vi "prepAO_focusalign.vi"(3 "srate":dbl=30000.0, 4 "waveforms":waveform(dbl)[][](array[waveform]), 5 "Device chans":T1(array[cluster]), 6 "bufferAO":i32) -> (0 "AOerrout":errorcluster[](array[cluster]), 1 "Terminal Name with Device Prefix":tag, 2 "aochanarrays":refnum<k21>[](array[refnum]))   [LabVIEW 2015]
uses:
  <vilib>/DAQmx/write.llb/DAQmx Write (Analog Wfm 1Chan NSamp).vi
  <vilib>/DAQmx/write.llb/DAQmx Write (Analog 1D Wfm NChan NSamp).vi
  <vilib>/DAQmx/create/channels.llb/DAQmx Create Channel (AO-Voltage-Basic).vi
  <vilib>/DAQmx/configure/timing.llb/DAQmx Timing (Sample Clock).vi
  <vilib>/DAQmx/miscellaneous.llb/DAQmx Fill In Error Info.vi
  <vilib>/DAQmx/configure/trigger.llb/DAQmx Start Trigger (Digital Edge).vi
panel:
  in  "error in 3":errorcluster caption="error in"
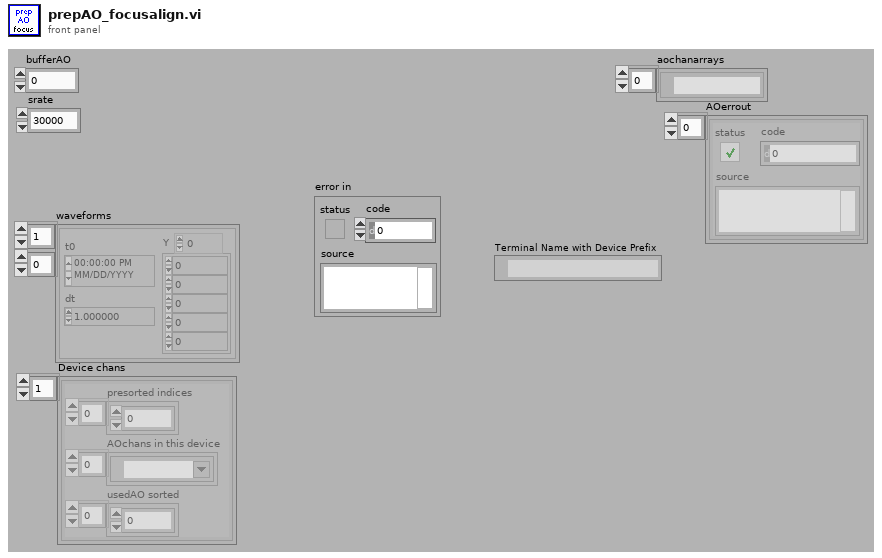
[diagram p1: front panel]
types:
  T1 = cluster{"presorted indices":i32[], "AOchans in this device":tag[], "usedAO sorted":i32[]}[]
  T2 = typedef "XYZStage.lvlib/XYZStage Configuration.ctl" = cluster{"VISA resource name":refnum<visa-resource-name>, "Timeout (3sec)":u32}
  T3 = cluster{"StageS":i32, "StageL":i32, "currmeas data dir":path, "image OD":u16, "contour OD":u16, "point OD":u16, "AOlines":tag[], "AIlines":tag[], "CI lines":tag[], "DO lines":tag[], "AO names":string[], "CI names":string[], "AI names":string[], "DO names":string[], "CIextensions":string[], "AIextensions":string[], "Voltage to Ygalvo":i32, "Voltage to Xgalvo":i32, "Voltage to patch":i32, "640 shutter":i32, "2P shutter":i32, "LT timestamp":u32, "Vp":i32, "Ip":i32, "camera trigger":i32, "master data dir":path, "voltage to Zpos":i32, "Vto2P":i32, "640 AO":i32, "488 AO":i32, "532 AO":i32, "640TTL":u32, "488TTL":u32, "532TTL":u32, "Device 1 sampleclock out":tag, "Device 1 Starttrigger out":tag, "Device 2 sampleclock in":tag, "Device 2 StartTrigger in ":tag, "2PODTTL":u32, "488 shutter":u32, "LCVR red":u32, "LCVR blue":u32, "Sutter Stage Config":T2}
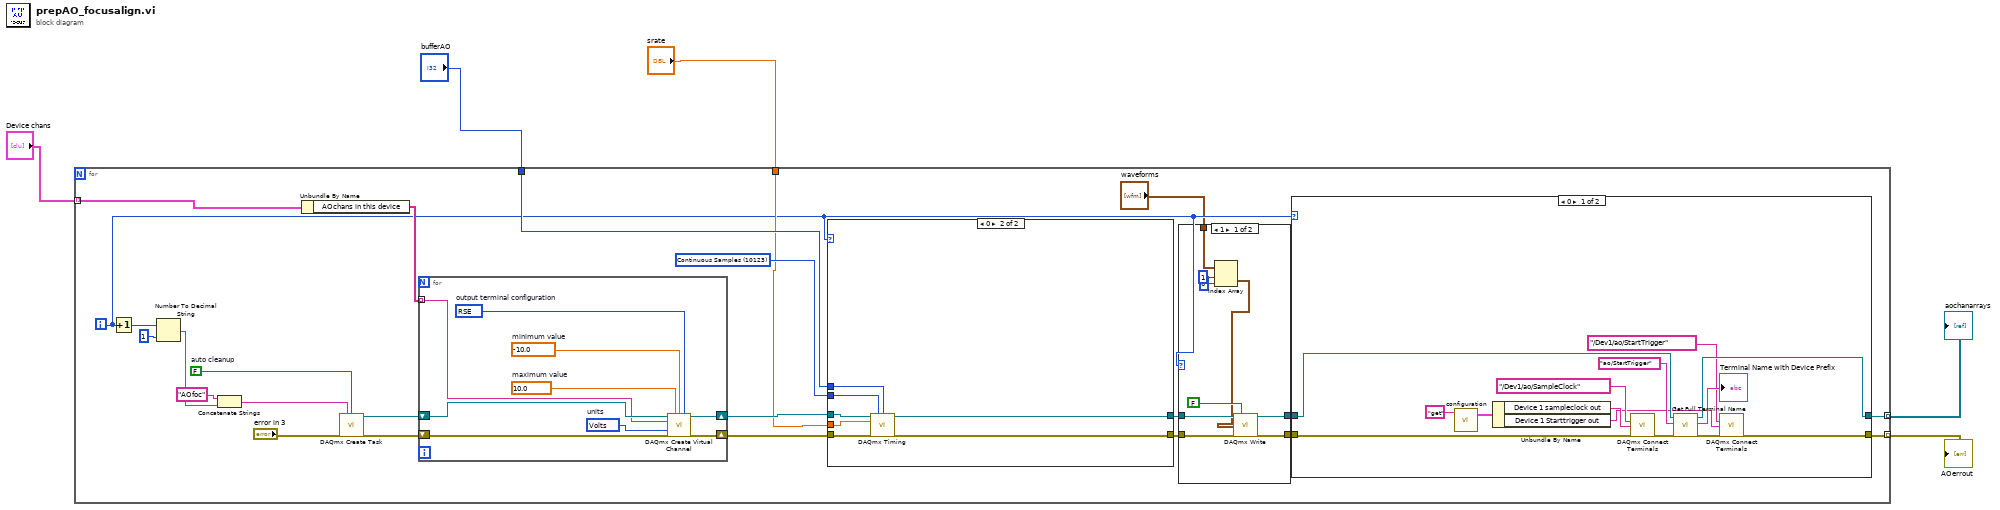
[diagram p0: block diagram]
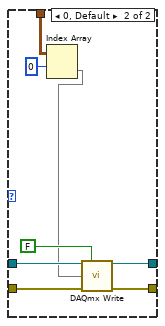
[diagram p2: hidden frame]
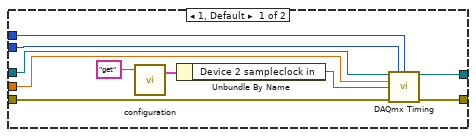
[diagram p3: hidden frame]
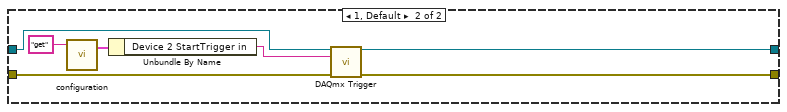
[diagram p4: hidden frame]
diagram:
  n1 = for {
    tunnel: "Device chans" -> [w23] mode=indexing
    tunnel: [w12] -> w5 mode=indexing
    tunnel: [w11] -> w4 mode=indexing
    tunnel: "bufferAO" -> [w9]
    tunnel: "srate" -> [w8]
    i -> [w7]
    w10 = 10123 items=["Finite Samples"=10178, "Continuous Samples"=10123, "Hardware Timed Single Point"=12522] ("sample mode")
    w27 = FALSE  # auto cleanup
    n2 = Increment(x=w7) -> (x+1=w20:i32)
    n3 = Number To Decimal String(number=w20, width (-)=i16 1) -> (decimal integer string=w19:string)
    n4 = Concatenate Strings("AOfoc" ("new task name"), w19) -> (w17:string)
    n5 = Unbundle By Name(w23) -> ("AOchans in this device"=w22:tag[])
    n6 = call <vilib>:"DAQmx Create Task.vi"("new task name"=w17, "auto cleanup"=w27, "error in"="error in 3") -> ("task out"=w28:refnum<k21>, "error out"=w29:errorcluster)  [unwired: 11 in]
    n7 = for {
      shift-right: [w87] -> w25
      shift-left: w28 -> [w89]
      shift-right: [w86] -> w24
      shift-left: w29 -> [w88]
      tunnel: w22 -> [w85] mode=indexing
      w93 = 10083 items=["Default"=-1, "RSE"=10083, "Differential"=10106, "Pseudodifferential"=12529]  # output terminal configuration
      w92 = 10348 items=["Volts"=10348, "From Custom Scale"=10065]  # units
      w91 = -10.0  # minimum value
      w90 = 10.0  # maximum value
      n8 = call-poly <vilib>:"DAQmx Create Virtual Channel.vi"("task in"=w89, "maximum value"=w90, "minimum value"=w91, "output terminal configuration"=w93, "physical channels"=w85, "units"=w92, "error in"=w88) -> ("task out"=w87:refnum<k21>, "error out"=w86:errorcluster)  [unwired: 7 in]
    }
    n9 = case shown="0" w7 {
      tunnel: w25 -> [w56 w63]
      tunnel: w24 -> [w55 w62]
      tunnel: w10 -> [w47 w61]
      tunnel: w8 -> [w54 w60]
      tunnel: w9 -> [w53 w59]
      tunnel: [w52 w58] -> w16
      tunnel: [w51 w57] -> w15
      frame 1, Default {
        n10 = call "configuration.vi"("command"="get") -> ("config out"=w49:T3)  [unwired: 2 in, 1 out]
        n11 = Unbundle By Name(w49) -> ("Device 2 sampleclock in"=w48:tag)
        n12 = call-poly <vilib>:"DAQmx Timing.vi"("task/channels in"=w56, "sample mode"=w47, "samples per channel"=w53, "rate"=w54, "source"=w48, "error in"=w55) -> ("task out"=w51:refnum<k21>, "error out"=w52:errorcluster)  [unwired: 1 in, 7 out]
      }
      frame 0 {
        n13 = call-poly <vilib>:"DAQmx Timing.vi"("task/channels in"=w63, "sample mode"=w61, "samples per channel"=w59, "rate"=w60, "error in"=w62) -> ("task out"=w57:refnum<k21>, "error out"=w58:errorcluster)  [unwired: 2 in, 7 out]
      }
    }
    n14 = case shown="1" w7 {
      tunnel: w16 -> [w37 w45]
      tunnel: w15 -> [w36 w44]
      tunnel: [w35 w43] -> w14
      tunnel: [w34 w42] -> w13
      tunnel: "waveforms" -> [w33 w41]
      frame 1 {
        n15 = Index Array(array=w33, index (row)=1, index (col)=0 ("disabled index (col)")) -> (element=w30:waveform(dbl))
        n16 = call-poly <vilib>:"DAQmx Write.vi"("task/channels in"=w36, "auto start"=FALSE, "data"=w30, "error in"=w37) -> ("task out"=w35:refnum<k21>, "error out"=w34:errorcluster)  [unwired: 9 in, 1 out]
      }
      frame 0, Default {
        n17 = Index Array(array=w41, index (row)=0) -> (element=w39:waveform(dbl)[])  [unwired: 1 in]
        n18 = call-poly <vilib>:"DAQmx Write.vi"("task/channels in"=w44, "auto start"=FALSE, "data"=w39, "error in"=w45) -> ("task out"=w43:refnum<k21>, "error out"=w42:errorcluster)  [unwired: 9 in, 1 out]
      }
    }
    n19 = case shown="0" w7 {
      tunnel: [w76 w84] -> w12
      tunnel: [w68 w83] -> w11
      tunnel: w13 -> [w72 w81]
      tunnel: w14 -> [w74 w82]
      frame 0 {
        n20 = call "configuration.vi"("command"="get") -> ("config out"=w67:T3)  [unwired: 2 in, 1 out]
        n21 = Unbundle By Name(w67) -> ("Device 1 sampleclock out"=w65:tag, "Device 1 Starttrigger out"=w64:tag)
        n22 = call <vilib>:"DAQmx Connect Terminals.vi"("source terminal"=tag "/Dev1/ao/SampleClock", "destination terminal"=w65, "error in"=w72) -> ("error out"=w71:errorcluster)  [unwired: 12 in]
        n23 = call "Get Full Terminal Name.vi"("error in"=w71, "Local Terminal Name"="ao/StartTrigger", "task/channels in"=w74) -> ("error out"=w69:errorcluster, "Terminal Name with Device Prefix"=→"Terminal Name with Device Prefix":tag, "task out"=w76:refnum<k21>)  [unwired: 6 in]
        n24 = call <vilib>:"DAQmx Connect Terminals.vi"("source terminal"=tag "/Dev1/ao/StartTrigger", "destination terminal"=w64, "error in"=w69) -> ("error out"=w68:errorcluster)  [unwired: 12 in]
      }
      frame 1, Default {
        n25 = call "configuration.vi"("command"="get") -> ("config out"=w79:T3)  [unwired: 2 in, 1 out]
        n26 = Unbundle By Name(w79) -> ("Device 2 StartTrigger in"=w78:tag)
        n27 = call-poly <vilib>:"DAQmx Trigger.vi"("task/channels in"=w82, "source"=w78, "error in"=w81) -> ("task out"=w84:refnum<k21>, "error out"=w83:errorcluster)  [unwired: 11 in]
      }
    }
  }
  "aochanarrays" <- w5
  "AOerrout" <- w4
